vi "Open.vi"(8 "error in (no error)":errorcluster, 10 "I2C Channel":u8, 11 "I2C Linx in":refnum<class "LinxI2C.lvclass">) -> (0 "error out":errorcluster, 3 "I2C Linx out":refnum<class "LinxI2C.lvclass">)   [LabVIEW 2014, in "LinxI2C.lvclass"]
doc: "Open the specified I2C channel. If the device has a single I2C master it is channel 0. If the device has more than one I2C master the logical first I2C master is channel 0, the next is channel 1, etc."
uses:
  LinxI2C.lvclass
  LinxI2C.lvclass/LinxI2C.ctl
  I2C.lvclass
  <vilib>/MakerHub/LINX/LMH-LINX.lvlib
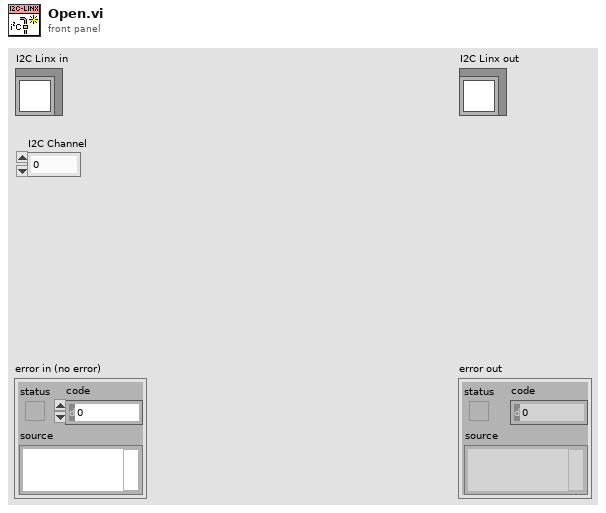
[diagram p1: front panel]
types:
  T1 = typedef "LMH-LINX.lvlib/LINX Ref.ctl" = cluster{"IO":T2, "Interface":T3, "LINX Device Config":T4}
  T2 = typedef "LMH-LINX.lvlib/Platform.ctl" = enum16{"Remote", "Local"}
  T3 = typedef "LMH-LINX.lvlib/Interface.ctl" = enum16{"Serial", "TCP"}
  T4 = typedef "LMH-LINX.lvlib/Device.lvlib/LINX Device Config.ctl" = cluster{"Interface":T3, "COM Port":refnum<visa-resource-name>, "TCP Configuration":T5, "Device Family":u8, "Device ID":u8, "Device Name":string, "TCP Ref":refnum<k5>, "Channels":T6}
  T5 = typedef "LMH-LINX.lvlib/Device.lvlib/TCP Config.ctl" = cluster{"IP Address":string, "Port":u16}
  T6 = typedef "LMH-LINX.lvlib/Channels.ctl" = cluster{"DI":u8[], "DO":u8[], "AI":u8[], "AO":u8[], "PWM":u8[], "QE":u8[], "UART":u8[], "I2C 2":u8[], "SPI":u8[], "CAN":u8[], "Servo":u8[], "AI Ref (V)":dbl, "AI Resolution (Bits)":u8, "AO Ref (V)":dbl, "AO Resolution (Bits)":u8}
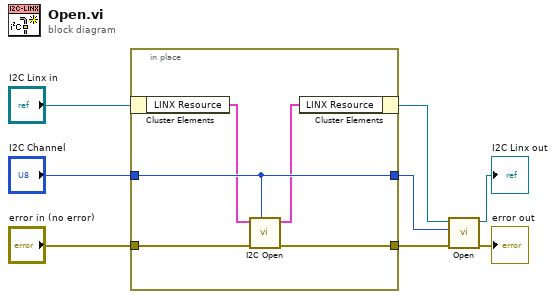
[diagram p0: block diagram]
diagram:
  n1 = in-place {
    in-place-border: "error in (no error)" -> [w13]
    in-place-border: [w12] -> w5
    in-place-border: "I2C Channel" -> [w11]
    in-place-border: [w11] -> w3
    n2 = in-place-cluster #1("I2C Linx in") -> ("LINX Resource"=w10:T1)
    n3 = call <vilib>:"I2C Open.vi"("I2C Channel (0)"=w11, "Error In"=w13, "LINX Resource"=w10) -> ("Error Out"=w12:errorcluster, "LINX Resource"=w9:T1)  [unwired: 7 in]
    n4 = in-place-cluster #1("LINX Resource"=w9) -> (w1:refnum<class "LinxI2C.lvclass">)
  }
  n5 = call-parent "Open.vi"("error in (no error)"=w5, "I2C Channel"=w3, "I2C in"=w1) -> ("error out"=→"error out":errorcluster, "I2C out"=→"I2C Linx out":refnum<class "LinxI2C.lvclass">)  [unwired: 7 in]
